vi "Ctor.vi"(8 "error in (no error)":errorcluster, 11 "Value Editor Base in":refnum<class "Value Editor Base.lvclass">) -> (0 "error out":errorcluster, 3 "Value Editor Base out":refnum<class "Value Editor Base.lvclass">)   [LabVIEW 2020, in "Value Editor Base.lvclass"]
uses:
  Value Editor Base.lvclass
  Ref Data.ctl
  Type Descriptor.ctl
  Terminal Direction.ctl
  Value Mode.ctl
  Special Terminal.ctl
  Terminal Mode.ctl
  Value Editor Base.lvclass/Value Editor Base.ctl
  <vilib>/IlluminatedG/IG OOPanel/OOPanel/ArrayPanel/ArrayPanel.lvclass
  FlexBlocks.lvlib
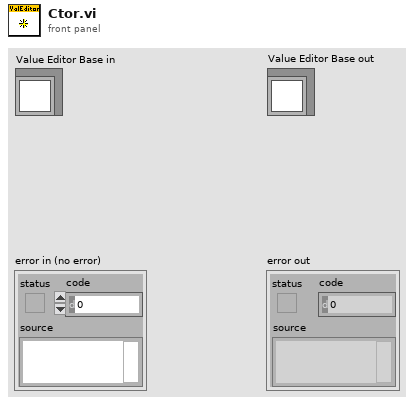
[diagram p1: front panel]
types:
  T1 = typedef "Value Editor Base.lvclass/Ref Data.ctl" = cluster{"Type Descriptor":T2, "Terminal Mode":T6, "Value":variant}
  T2 = typedef "FlexBlocks.lvlib/Type Descriptor.ctl" = cluster{"Name":string, "Direction":T3, "Default":variant, "Min":variant, "Max":variant, "Step":variant, "Value Mode":T4, "Required":bool, "Connpane Index":i32, "Special Terminal":T5, "Color":u32, "Options":string[], "Type String":string, "Sort":i32, "Item Path":path}
  T3 = typedef "FlexBlocks.lvlib/Terminal Direction.ctl" = enum16{"Sink", "Source"}
  T4 = typedef "FlexBlocks.lvlib/Value Mode.ctl" = enum16{"Normal", "Range", "Select"}
  T5 = typedef "FlexBlocks.lvlib/Special Terminal.ctl" = enum16{"None", "Action", "Init", "Tag", "State in", "State out", "Error"}
  T6 = typedef "FlexBlocks.lvlib/Terminal Mode.ctl" = enum16{"Channel", "Config", "Value", "Control Ref"}
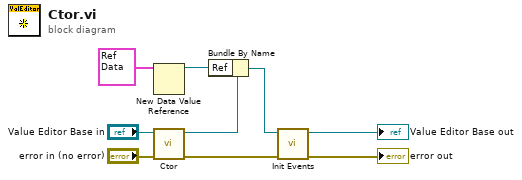
[diagram p0: block diagram]
diagram:
  n1 = New Data Value Reference(data value=T1 {"Type Descriptor"={"Name"="", "Direction"=enum."Sink", "Default"=variant, "Min"=variant, "Max"=variant, "Step"=variant, "Value Mode"=enum."Normal", "Required"=FALSE, "Connpane Index"=0, "Special Terminal"=enum."None", "Color"=0, "Options"=[], "Type String"="", "Sort"=0, "Item Path"=path ""}, "Terminal Mode"=enum."Channel", "Value"=variant} ("Ref Data")) -> (data value reference=w5:refnum<data-value>)  [unwired: 1 in, 1 out]
  n2 = call-parent "Ctor.vi"("error in (no error)"="error in (no error)", "ArrayPanel in"="Value Editor Base in") -> ("error out"=w4:errorcluster, "ArrayPanel out"=w6:refnum<class "Value Editor Base.lvclass">)  [unwired: 8 in]
  n3 = Bundle By Name(cluster=w6, "Ref"=w5) -> (w3:refnum<class "Value Editor Base.lvclass">)
  n4 = call "Init Events.vi"("error in (no error)"=w4, "Value Editor Base in"=w3) -> ("error out"=→"error out":errorcluster, "Value Editor Base out"=→"Value Editor Base out":refnum<class "Value Editor Base.lvclass">)  [unwired: 8 in]
